vi "AalborgMFC.vi"(7 "Value to Output":dbl format="%.2f", 8 "Ch Description":T1={"Ch Name"="GRC-A:N2-1:SP(%)", "Type"="AalborgMFC", "Function"=enum."Analogue Output", "Ch State"=enum."On", "Calibration type"="Raw", "A"=0.0, "B"=0.0, "C"=0.0, "D"=0.0, "Comments"="!ASYNC", "Address"={"Main"=170, "Ch."=0, "Sub"=0, "Port Name"="tcp://192.168.126.152:10001/"}, "String"="Front Panel", "Duty"=65535} {"Duty" format="%016b"; "D" format="%#_5g"; "C" format="%#_5g"; "B" format="%#_5g"; "A" format="%#_5g"}) -> (0 "Scan comment":string, 1 "Output":dbl=nan format="%.3f", 3 "HelpText":string="Analogue Input: Reads flowrate\nAnalogue Output: Sets digital control, sets setpoint, puts valve in auto\nNegative demand will ForceValveClosed\nDigital Output: 0-forceClosed, else-Automatic")   [LabVIEW 2021]
uses:
  ADAM Client/Sub VIs/ADAM Controls/Ch_description_ADAM.ctl
  ADAM Client/Sub VIs/ADAM Controls/Module_type_ADAM.ctl
  ADAM Client/Sub VIs/ADAM Controls/Function_ADAM.ctl
  ADAM Client/Sub VIs/ADAM Controls/Channel_State.ctl
  ADAM Client/Sub VIs/ADAM Controls/Calib_type_ADAM.ctl
  ADAM Client/Sub VIs/ADAM Controls/Address.ctl
  subVIs/AalborgDFCCommand.ctl
panel:
  out "execTime 3":dbl caption="Avg Execution Time" format="%_3ps"
  out "nCalls":dbl
  out "execTime 2":dbl caption="Execution Time" format="%_3ps"
  out "GoodComms":bool
  # "VI to control Aalborg Digital Mass Flow Controller"
  # "https://www.aalborg.com/index.php/main_page/product_overview/id_product_overview/24"
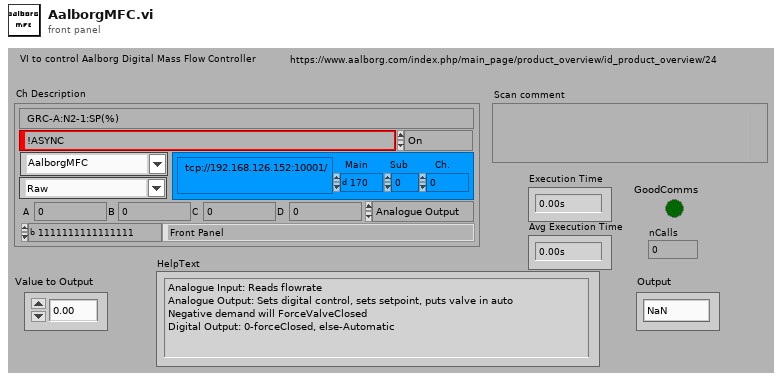
[diagram p1: front panel]
types:
  T1 = typedef "Ch_description_ADAM.ctl" = cluster{"Ch Name":string, "Type":T2, "Function":T3, "Ch State":T4, "Calibration type":T5, "A":dbl, "B":dbl, "C":dbl, "D":dbl, "Comments":string, "Address":T6, "String":string, "Duty":u16}
  T2 = typedef "Module_type_ADAM.ctl" = string
  T3 = typedef "Function_ADAM.ctl" = enum16{"Analogue Input", "Digital Input", "Event counter", "Event rate", "Analogue Output", "Digital Output", "Relay Output"}
  T4 = typedef "Channel_State.ctl" = enum16{"On", "Off", "Always On", "Always Off"}
  T5 = typedef "Calib_type_ADAM.ctl" = string
  T6 = typedef "Address.ctl" = cluster{"Main":i32, "Ch.":i32, "Sub":i32, "Port Name":string}
  T7 = typedef "AalborgDFCCommand.ctl" = string
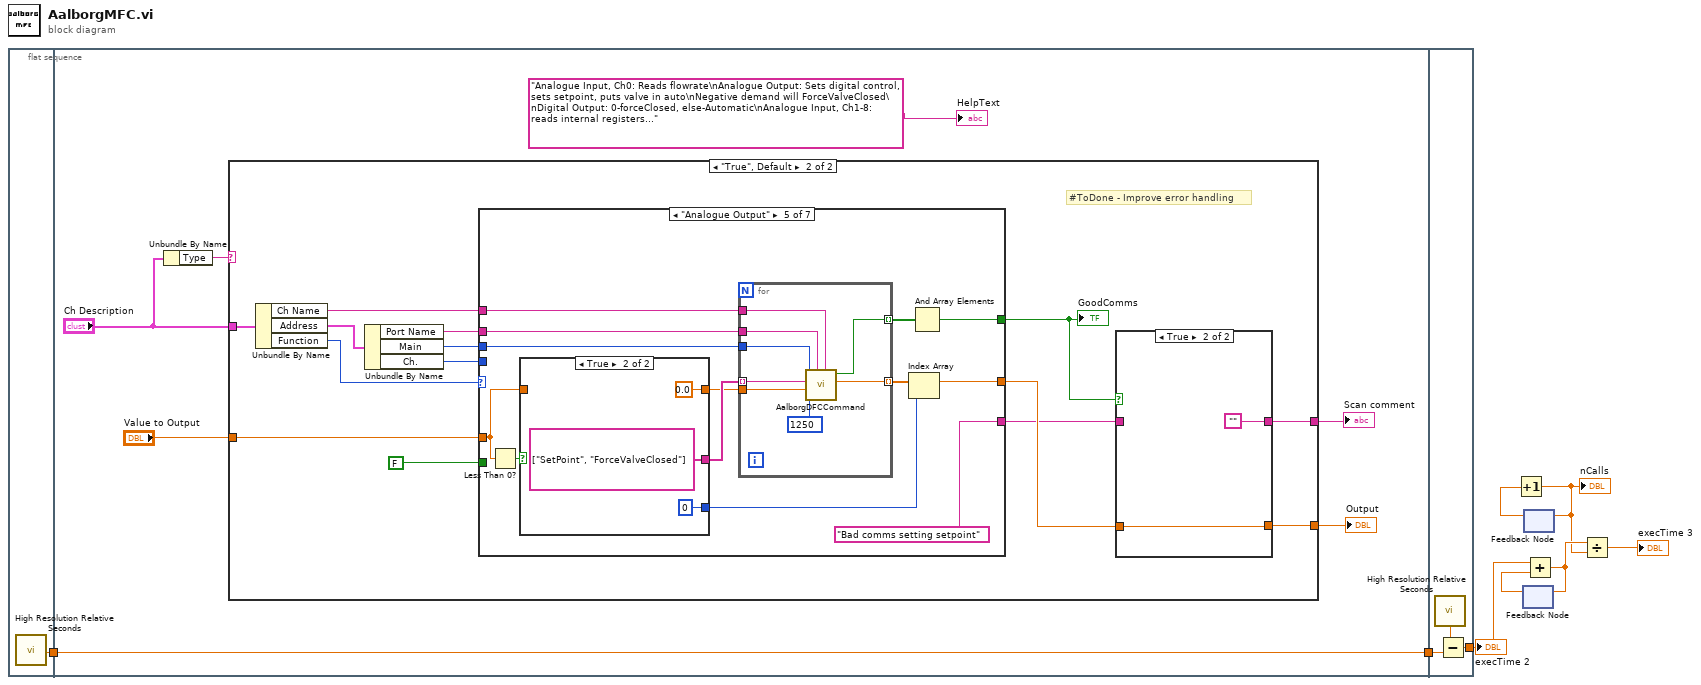
[diagram p0: block diagram]
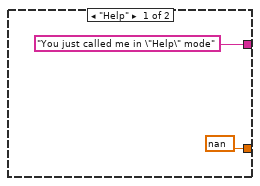
[diagram p2: hidden frame]
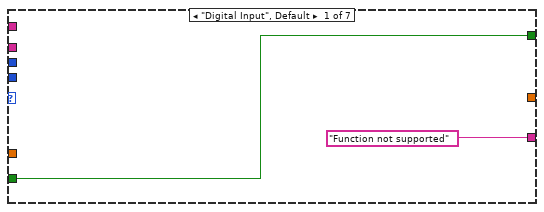
[diagram p3: hidden frame]
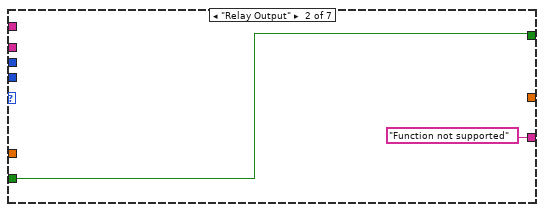
[diagram p4: hidden frame]
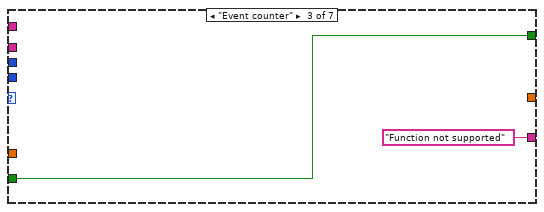
[diagram p5: hidden frame]
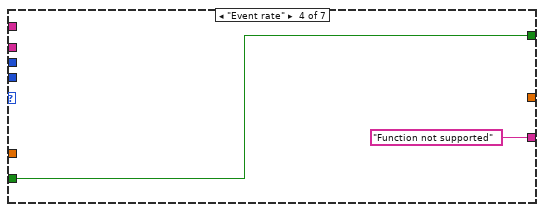
[diagram p6: hidden frame]
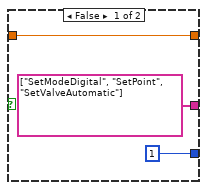
[diagram p7: hidden frame]
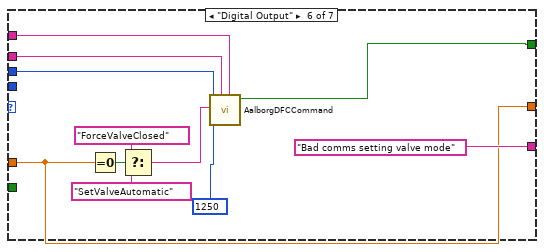
[diagram p8: hidden frame]
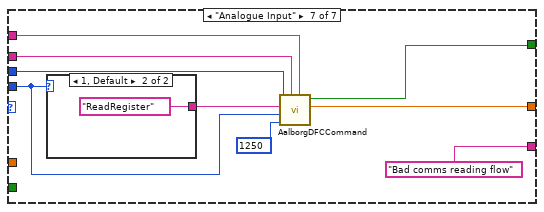
[diagram p9: hidden frame]
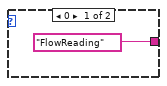
[diagram p10: hidden frame]
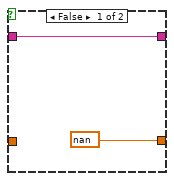
[diagram p11: hidden frame]
diagram:
  n1 = flat-sequence {
    tunnel: [w9] -> w8
    tunnel: w8 -> [w16]
    tunnel: [w16] -> w7
    tunnel: w7 -> [w95]
    tunnel: [w94] -> w2
    frame #0 {
      n2 = call <vilib>:"High Resolution Relative Seconds.vi"() -> ("relative seconds"=w9:dbl)
    }
    frame #1 {
      n3 = Unbundle By Name("Ch Description") -> ("Type"=w14:T2)
      n4 = case shown="\"True\", Default" w14 {
        tunnel: ["You just called me in \"Help\" mode" w31] -> w11
        tunnel: [nan ("t") w30] -> w12
        tunnel: "Ch Description" -> [_ w28]
        tunnel: "Value to Output" -> [_ w23]
        frame "Help" {
        }
        frame "True", Default {
          # "#ToDone - Improve error handling"
          n5 = Unbundle By Name(w28) -> ("Ch Name"=w24:string, "Address"=w32:T6, "Function"=w27:T3)
          n6 = Unbundle By Name(w32) -> ("Port Name"=w26:string, "Main"=w29:i32, "Ch."=w19:i32)
          n7 = case shown="\"Analogue Output\"" w27 {
            tunnel: w29 -> [_ _ _ _ w52 w77 w86]
            tunnel: w26 -> [_ _ _ _ w53 w78 w87]
            tunnel: [_ _ _ _ w48 w68 w84] -> w25
            tunnel: w24 -> [_ _ _ _ w51 w76 w83]
            tunnel: w23 -> [_ _ _ _ w43 w68 _]
            tunnel: [w34 w36 w38 w40 w46 w71 w82] -> w22
            tunnel: FALSE -> [w34 w36 w38 w40 _ _ _]
            tunnel: ["Function not supported" "Function not supported" "Function not supported" "Function not supported" "Bad comms setting setpoint" "Bad comms setting valve mode" "Bad comms reading flow"] -> w20
            tunnel: w19 -> [_ _ _ _ _ _ w79]
            frame "Digital Input", Default {
            }
            frame "Relay Output" {
            }
            frame "Event counter" {
            }
            frame "Event rate" {
            }
            frame "Analogue Output" {
              n8 = Less Than 0?(x=w43) -> (x < 0?=w44:bool)
              n9 = case shown="True" w44 {
                tunnel: [T7[] ["SetModeDigital", "SetPoint", "SetValveAutomatic"] T7[] ["SetPoint", "ForceValveClosed"]] -> w49
                tunnel: w43 -> [w55 _]
                tunnel: [w55 0.0 ("Value to Output")] -> w42
                tunnel: [1 ("index") 0 ("index")] -> w41
                frame False {
                }
                frame True {
                }
              }
              n10 = for {
                tunnel: w53 -> [w67]
                tunnel: w52 -> [w66]
                tunnel: w49 -> [w65] mode=indexing
                tunnel: w51 -> [w64]
                tunnel: w42 -> [w62]
                tunnel: [w61] -> w50 mode=indexing
                tunnel: [w60] -> w47 mode=indexing
                n11 = call "AalborgDFCCommand.vi"("Channel Name"=w64, "Port Name"=w67, "Timeout/ms"=u32 1250, "Numeric Value"=w62, "AalborgDFCCommand"=w65, "Address"=w66) -> ("Numeric Reply"=w61:dbl, "OK"=w60:bool)  [unwired: 1 in, 2 out]
              }
              n12 = Index Array(array=w50, index=w41) -> (element=w48:dbl)
              n13 = And Array Elements(Boolean array=w47) -> (logical AND=w46:bool)
            }
            frame "Digital Output" {
              n14 = Equal To 0?(x=w68) -> (x = 0?=w75:bool)
              n15 = Select(t=T7 "ForceValveClosed" ("AalborgDFCCommand"), s=w75, f=T7 "SetValveAutomatic" ("AalborgDFCCommand")) -> (s? t:f=w72:T7)
              n16 = call "AalborgDFCCommand.vi"("Channel Name"=w76, "Port Name"=w78, "Timeout/ms"=u32 1250, "AalborgDFCCommand"=w72, "Address"=w77) -> ("OK"=w71:bool)  [unwired: 2 in, 3 out]
            }
            frame "Analogue Input" {
              n17 = case shown="1, Default" w79 {
                tunnel: [T7 "FlowReading" ("AalborgDFCCommand") T7 "ReadRegister" ("AalborgDFCCommand")] -> w85
                frame 0 {
                }
                frame 1, Default {
                }
              }
              n18 = call "AalborgDFCCommand.vi"("Channel Name"=w83, "Port Name"=w87, "Timeout/ms"=u32 1250, "Numeric Value"=w79, "AalborgDFCCommand"=w85, "Address"=w86) -> ("Numeric Reply"=w84:dbl, "OK"=w82:bool)  [unwired: 1 in, 2 out]
            }
          }
          "GoodComms" <- w22
          n19 = case shown="True" w22 {
            tunnel: [w90 ""] -> w31
            tunnel: [nan ("t") w92] -> w30
            tunnel: w25 -> [_ w92]
            tunnel: w20 -> [w90 _]
            frame False {
            }
            frame True {
            }
          }
        }
      }
      "Output" <- w12
      "Scan comment" <- w11
      "HelpText" <- "Analogue Input, Ch0: Reads flowrate\nAnalogue Output: Sets digital control, sets setpoint, puts valve in auto\nNegative demand will ForceValveClosed\nDigital Output: 0-forceClosed, else-Automatic\nAnalogue Input, Ch1-8: reads internal registers..."
    }
    frame #2 {
      n20 = call <vilib>:"High Resolution Relative Seconds.vi"() -> ("relative seconds"=w96:dbl)
      n21 = Subtract(x=w96, y=w95) -> (x-y=w94:dbl)
    }
  }
  n22 = feedback #1() -> (w3:dbl)  [unwired: 1 in]
  n23 = feedback #2() -> (w4:dbl)  [unwired: 1 in]
  n24 = Increment(x=w4) -> (x+1=w5:dbl)
  "nCalls" <- w5
  n25 = feedback-in #2(w5) -> ()
  n26 = Add(x=w2, y=w3) -> (x+y=w6:dbl)
  n27 = feedback-in #1(w6) -> ()
  n28 = Divide(x=w6, y=w5) -> (x/y=→"execTime 3":dbl)
  "execTime 2" <- w2
